vi "IsHalted.vi"(8 "error in (no error)":errorcluster, 11 "FHPP in":refnum<class "FHPP.lvclass">) -> (0 "error out":errorcluster, 3 "FHPP out":refnum<class "FHPP.lvclass">)   [LabVIEW 2022 SP3, in "FHPP.lvclass"]
uses:
  FHPP.lvclass
  FHPP.lvclass/FHPP.ctl
panel:
  out "IsHalted":bool
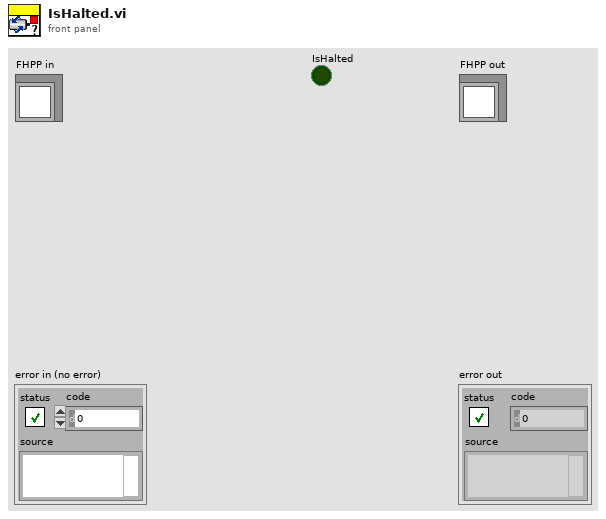
[diagram p1: front panel]
types:
  T1 = typedef "FHPP.lvclass/SPOS.ctl" = cluster{"Halt":bool, "Ack Start":bool, "Motion Complete":bool, "Ack Teach":bool, "Axis Moving":bool, "Drag Error":bool, "Standstill Control":bool, "Axis Referenced":bool}
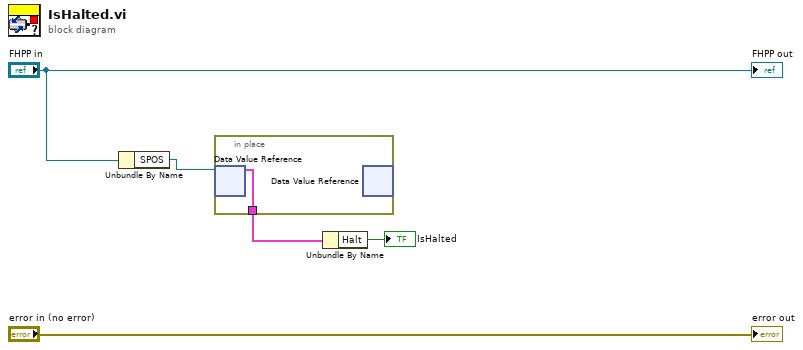
[diagram p0: block diagram]
diagram:
  n1 = Unbundle By Name("FHPP in") -> ("SPOS"=w3:refnum<data-value>)
  n2 = in-place {
    in-place-border: [w6] -> w2
    n3 = in-place-dvr #1(w3) -> (w6:T1)  [unwired: 1 out]
    n4 = in-place-dvr #1() -> ()  [unwired: 1 in, 2 out]
  }
  n5 = Unbundle By Name(w2) -> ("Halt"=→"IsHalted":bool)
  "error out" <- "error in (no error)"
  "FHPP out" <- "FHPP in"
